vi "Check Expiration.vi"(0 "Charact Result Accessor in":refnum<class "Charact Result Accessor.lvclass">, 11 "error in":errorcluster) -> (4 "Charact Result Accessor out":refnum<class "Charact Result Accessor.lvclass">, 6 "Expired?":bool, 15 "error out":errorcluster)   [LabVIEW 2023, in "RFFixtureCharact.RFPM.lvlib" / "Charact Result Accessor.lvclass"]
uses:
  Charact Result Accessor.lvclass
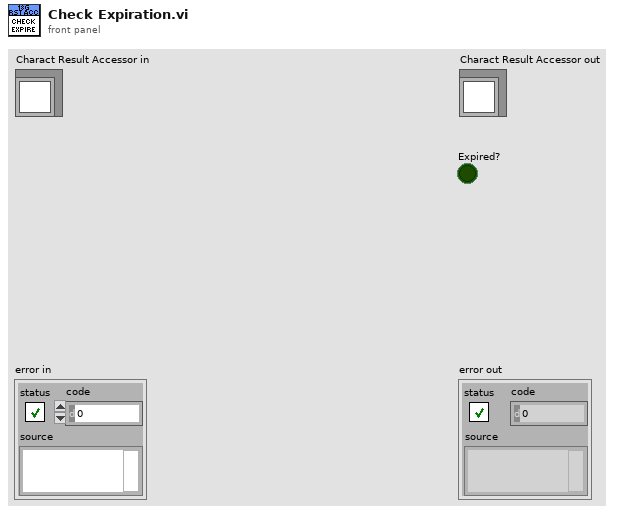
[diagram p1: front panel]
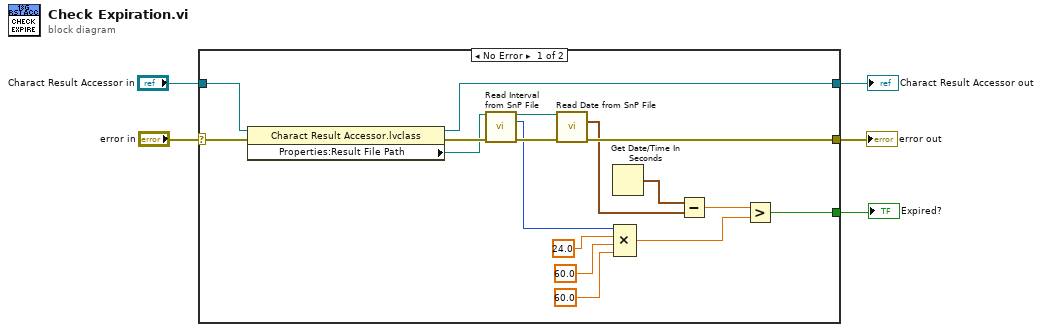
[diagram p0: block diagram]
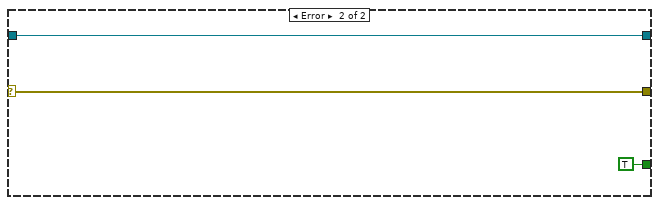
[diagram p2: hidden frame]
diagram:
  n1 = case shown="No Error" "error in" {
    selector: "error in" -> [w19 w25]
    tunnel: [w20 w25] -> w4
    tunnel: [w17 w24] -> w3
    tunnel: "Charact Result Accessor in" -> [w18 w24]
    tunnel: [w6 TRUE] -> w1
    frame No Error {
      n2 = property class="Charact Result Accessor.lvclass"(reference=w18, error in=w19) -> (reference out=w17:refnum<class "Charact Result Accessor.lvclass">, error out=w16:errorcluster, "Properties:Result File Path"=w15:path)
      n3 = call "Read Interval from SnP File.vi"("Result File Path In"=w15, "error in"=w16) -> ("Result File Path Out"=w21:path, "Interval"=w8:i32, "error out"=w22:errorcluster)  [unwired: 11 in]
      n4 = call "Read Date from SnP File.vi"("Result File Path"=w21, "error in (no error)"=w22) -> ("Path Charact Date"=w7:timestamp, "error out"=w20:errorcluster)  [unwired: 11 in, 1 out]
      n5 = Get Date/Time In Seconds() -> (seconds since 1Jan1904=w14:timestamp)
      n6 = Compound Arithmetic op=MULTIPLY(w8, 24.0 ("value"), 60.0 ("value"), 60.0 ("value")) -> (w9:dbl)
      n7 = Subtract(x=w14, y=w7) -> (x-y=w10:dbl)
      n8 = Greater?(x=w10, y=w9) -> (0:w6:bool)
    }
    frame Error {
    }
  }
  "error out" <- w4
  "Charact Result Accessor out" <- w3
  "Expired?" <- w1
